vi "Interactive_Test_Panel_BackgroundVI.vi"() -> ()   [LabVIEW 2014]
uses:
  <vilib>/Motion/plugins/PluginFramework/nismSDIFramework.SetFrameworkMode.single.vi
  <vilib>/Motion/Express/_s/nimc.ex.clearFaults.clearFaults.axis.vi
  <vilib>/Motion/BlockNode/FB.NIMotion.xnode
  <vilib>/Motion/plugins/Delta SDI Plug-in/Template SoftMotion Drive Interface Plug-in Class.lvclass
panel:
  in  "stop":bool
  in  "Motion Resource":refnum<k21>="Axis 1"
  out "error out":errorcluster
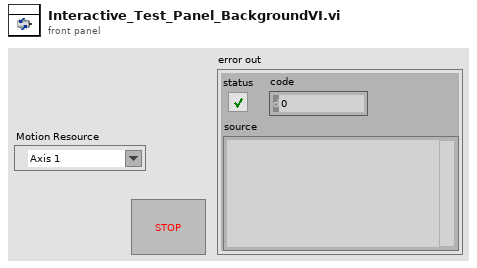
[diagram p1: front panel]
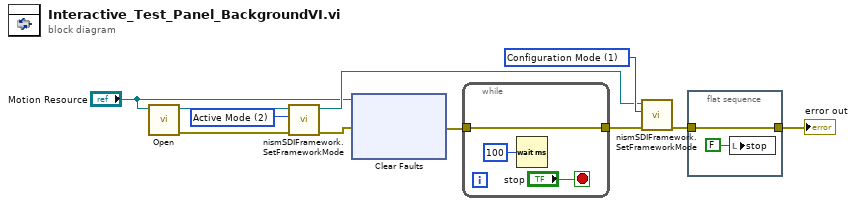
[diagram p0: block diagram]
diagram:
  w10 = 1 items=["Configuration Mode"=1, "Active Mode"=2] ("mode (Active Mode)")
  w11 = 2 items=["Configuration Mode"=1, "Active Mode"=2] ("mode (Active Mode)")
  n1 = call <vilib>:"Open.vi"("Axis"="Motion Resource") -> ("error out"=w3:errorcluster, "Base Axis Out"=w4:refnum<class "nismPluginAxisBaseClass.lvclass">)  [unwired: 9 in]
  n2 = call-poly <vilib>:"nismSDIFramework.SetFrameworkMode.vi"("error in (no error)"=w3, "mode (Active Mode)"=w11, "Base Axis In"=w4) -> ("error out"=w7:errorcluster, "Base Axis Out"=w8:refnum<class "nismPluginAxisBaseClass.lvclass">)  [unwired: 7 in]
  n3 = xnode ("Clear Faults")("resource"="Motion Resource", "error in"=w7) -> ("error out"=w1:errorcluster)  [unwired: 1 out]
  n4 = while {
    tunnel: w1 -> [w13]
    tunnel: [w13] -> w9
    stop <- "stop" stop-if-true
    n5 = Wait (ms)(milliseconds to wait=u32 100) -> ()  [unwired: 1 out]
  }
  n6 = call-poly <vilib>:"nismSDIFramework.SetFrameworkMode.vi"("error in (no error)"=w9, "mode (Active Mode)"=w10, "Base Axis In"=w8) -> ("error out"=w6:errorcluster)  [unwired: 7 in, 1 out]
  n7 = flat-sequence {
    tunnel: w6 -> [w16]
    tunnel: [w16] -> w5
    frame #0 {
      n8 = local write "stop"(FALSE ("stop")) -> ()
    }
  }
  "error out" <- w5
